vi "ADC Get Capabilities.vi"(7 "Initialize HW? (False)":bool, 8 "error in":errorcluster, 10 "parameters":T1, 11 "adc session in":T4={"niScope"={"channel cfg"=[], "sessions"=[], "multi cards"=FALSE, "channels"=0, "type"=enum."n/a", "memory [B/chn]"=0, "ext. clock [Hz]"=0.0, "samples count"=0, "use streaming"=FALSE, "proc setup"={"packet size [smpl]"=0, "current timeout [s]"=0.0, "blk2blk timeout [s]"=0.0, "event time"=timestamp(0 s since 1904-01-01), "temp sampl T [s]"=0.0, "data queue"=refnum, "stop notifier"=refnum, "proc ref"=refnum}, "sample width [B]"=0, "ranges [V]"=[], "trigger setup"={"coupling"=1, "level [V]"=0.0, "slope"=0, "mode"=enum."Immediate"}, "fs [Hz]"=0.0, "bitres [bit]"=0}, "3458A"={"channels"=[], "sync unit"={"VISA"="", "type"=enum."Picotest U6200A"}, "awg unit"={"type"=enum."Agilent 331xxA to 332xxA", "VISA"="", "enable 10MHz ref"=FALSE}, "sync mode"=enum."MASTER-SLAVE, MASTER clocked by TIMER", "streaming mode"=FALSE, "idn mode"=enum."Auto", "sampling mode"=enum."DCV", "Ts [s]"=0.0, "sample memory [B]"=0, "proc setup"={"channel id"=0, "packet size [smpl]"=0, "current timeout [s]"=0.0, "blk2blk timeout [s]"=0.0, "event time"=timestamp(0 s since 1904-01-01), "stop notifier"=refnum, "data queues"=[], "proc refs"=[], "bus semaphore"=refnum}, "sample size [B]"=0, "sample count"=0, "aux data"={"channel id"=0, "valid?"=[], "gain [V]"=[], "timestamp [s]"=[], "Ts [s]"=0.0, "abs timestamp"=timestamp(0 s since 1904-01-01), "t [deg C]"=[]}, "ranges [V]"=[], "aperture [s]"=0.0, "LEVEL trigger"={"edge"=enum."POS", "level [V]"=0.0, "coupling"=enum."DC"}, "trigger mode"=enum."AUTO", "measure temp.?"=FALSE, "disp mesages"=[], "shared bus?"=FALSE, "disable display?"=FALSE, "aper mode"=enum."Manual", "aper rules"=[]}, "dsdll"={"dsdll"={"dsdll path"=path "", "dsdll handle"=[], "output devices"=[], "capture devices"=[]}, "channels"=0, "device id"=0, "channel idns"=[], "proc setup"={"packet size [smpl]"=0, "current timeout [s]"=0.0, "blk2blk timeout [s]"=0.0, "event time"=timestamp(0 s since 1904-01-01), "data queue"=refnum, "stop notifier"=refnum, "proc ref"=refnum}, "samples count"=0, "fs [Hz]"=0.0}, "type"=enum."niScope", "channel idn str"=[], "aux instr idn str"=[], "modified?"=FALSE, "simadc"={"channels"=[], "range [V]"=0.0, "Ts step [s]"=0.0, "time [s]"=0.0, "fs [Hz]"=0.0, "count"=0, "smpl offset"=0, "set count"=0, "bit res"=0}, "force rst?"=FALSE, "exit mode"=enum."Immediate reset", "exit dly"=0.0, "exit tmr"=timestamp(0 s since 1904-01-01), "busy?"=FALSE, "accessed?"=FALSE, "QuADC session"={"channel cfg"=[], "sessions"=[], "multi cards"=FALSE, "channels"=0, "type"=enum."n/a", "memory [B/chn]"=0, "ext. clock [Hz]"=0.0, "samples count"=0, "use streaming"=FALSE, "proc setup"={"packet size [smpl]"=0, "current timeout [s]"=0.0, "blk2blk timeout [s]"=0.0, "event time"=timestamp(0 s since 1904-01-01), "temp sampl T [s]"=0.0, "data queue"=refnum, "stop notifier"=refnum, "proc ref"=refnum}, "sample width [B]"=0, "ranges [V]"=[], "trigger setup"={"coupling"=1, "level [V]"=0.0, "slope"=0, "mode"=enum."Immediate"}, "fs [Hz]"=0.0, "bitres [bit]"=0}} {"QuADC session"."trigger setup"."level [V]" format="%.2f"; "QuADC session"."trigger setup"."coupling" items=["AC"=0, "DC"=1, "HF Reject"=3, "LF Reject"=4, "AC Plus HF Reject"=1001]; "QuADC session"."channel cfg"."Clock fr. (Hz)" min=0.0 format="%#_9p"; "QuADC session"."channel cfg"."Number of JJ" min=1; "QuADC session"."channel cfg"."Range [Vpk]" min=0.0; "QuADC session"."channel cfg"."Channel" min=0; "3458A"."channels"."Range [Vpk]" min=0.0; "niScope"."trigger setup"."level [V]" format="%.2f"; "niScope"."trigger setup"."coupling" items=["AC"=0, "DC"=1, "HF Reject"=3, "LF Reject"=4, "AC Plus HF Reject"=1001]; "niScope"."channel cfg"."Range [Vpk]" min=0.0; "niScope"."channel cfg"."Channel" min=0}) -> (0 "error out":errorcluster, 2 "capabilities":T2, 3 "adc session out":T4={"niScope"={"channel cfg"=[], "sessions"=[], "multi cards"=FALSE, "channels"=0, "type"=enum."n/a", "memory [B/chn]"=0, "ext. clock [Hz]"=0.0, "samples count"=0, "use streaming"=FALSE, "proc setup"={"packet size [smpl]"=0, "current timeout [s]"=0.0, "blk2blk timeout [s]"=0.0, "event time"=timestamp(0 s since 1904-01-01), "temp sampl T [s]"=0.0, "data queue"=refnum, "stop notifier"=refnum, "proc ref"=refnum}, "sample width [B]"=0, "ranges [V]"=[], "trigger setup"={"coupling"=1, "level [V]"=0.0, "slope"=0, "mode"=enum."Immediate"}, "fs [Hz]"=0.0, "bitres [bit]"=0}, "3458A"={"channels"=[], "sync unit"={"VISA"="", "type"=enum."Picotest U6200A"}, "awg unit"={"type"=enum."Agilent 331xxA to 332xxA", "VISA"="", "enable 10MHz ref"=FALSE}, "sync mode"=enum."MASTER-SLAVE, MASTER clocked by TIMER", "streaming mode"=FALSE, "idn mode"=enum."Auto", "sampling mode"=enum."DCV", "Ts [s]"=0.0, "sample memory [B]"=0, "proc setup"={"channel id"=0, "packet size [smpl]"=0, "current timeout [s]"=0.0, "blk2blk timeout [s]"=0.0, "event time"=timestamp(0 s since 1904-01-01), "stop notifier"=refnum, "data queues"=[], "proc refs"=[], "bus semaphore"=refnum}, "sample size [B]"=0, "sample count"=0, "aux data"={"channel id"=0, "valid?"=[], "gain [V]"=[], "timestamp [s]"=[], "Ts [s]"=0.0, "abs timestamp"=timestamp(0 s since 1904-01-01), "t [deg C]"=[]}, "ranges [V]"=[], "aperture [s]"=0.0, "LEVEL trigger"={"edge"=enum."POS", "level [V]"=0.0, "coupling"=enum."DC"}, "trigger mode"=enum."AUTO", "measure temp.?"=FALSE, "disp mesages"=[], "shared bus?"=FALSE, "disable display?"=FALSE, "aper mode"=enum."Manual", "aper rules"=[]}, "dsdll"={"dsdll"={"dsdll path"=path "", "dsdll handle"=[], "output devices"=[], "capture devices"=[]}, "channels"=0, "device id"=0, "channel idns"=[], "proc setup"={"packet size [smpl]"=0, "current timeout [s]"=0.0, "blk2blk timeout [s]"=0.0, "event time"=timestamp(0 s since 1904-01-01), "data queue"=refnum, "stop notifier"=refnum, "proc ref"=refnum}, "samples count"=0, "fs [Hz]"=0.0}, "type"=enum."niScope", "channel idn str"=[], "aux instr idn str"=[], "modified?"=FALSE, "simadc"={"channels"=[], "range [V]"=0.0, "Ts step [s]"=0.0, "time [s]"=0.0, "fs [Hz]"=0.0, "count"=0, "smpl offset"=0, "set count"=0, "bit res"=0}, "force rst?"=FALSE, "exit mode"=enum."Immediate reset", "exit dly"=0.0, "exit tmr"=timestamp(0 s since 1904-01-01), "busy?"=FALSE, "accessed?"=FALSE, "QuADC session"={"channel cfg"=[], "sessions"=[], "multi cards"=FALSE, "channels"=0, "type"=enum."n/a", "memory [B/chn]"=0, "ext. clock [Hz]"=0.0, "samples count"=0, "use streaming"=FALSE, "proc setup"={"packet size [smpl]"=0, "current timeout [s]"=0.0, "blk2blk timeout [s]"=0.0, "event time"=timestamp(0 s since 1904-01-01), "temp sampl T [s]"=0.0, "data queue"=refnum, "stop notifier"=refnum, "proc ref"=refnum}, "sample width [B]"=0, "ranges [V]"=[], "trigger setup"={"coupling"=1, "level [V]"=0.0, "slope"=0, "mode"=enum."Immediate"}, "fs [Hz]"=0.0, "bitres [bit]"=0}} {"QuADC session"."trigger setup"."level [V]" format="%.2f"; "QuADC session"."trigger setup"."coupling" items=["AC"=0, "DC"=1, "HF Reject"=3, "LF Reject"=4, "AC Plus HF Reject"=1001]; "QuADC session"."channel cfg"."Clock fr. (Hz)" min=0.0 format="%#_9p"; "QuADC session"."channel cfg"."Number of JJ" min=1; "QuADC session"."channel cfg"."Range [Vpk]" min=0.0; "QuADC session"."channel cfg"."Channel" min=0; "3458A"."channels"."Range [Vpk]" min=0.0; "niScope"."trigger setup"."level [V]" format="%.2f"; "niScope"."trigger setup"."coupling" items=["AC"=0, "DC"=1, "HF Reject"=3, "LF Reject"=4, "AC Plus HF Reject"=1001]; "niScope"."channel cfg"."Range [Vpk]" min=0.0; "niScope"."channel cfg"."Channel" min=0})   [LabVIEW 2018]
doc: "This VI returns cluster of capabilities for selected HW. Note that to make it work the session must be either live (opened) or at least were opened and closed so the HW paramter data are in the session. Alternatively use option 'initialize HW'. That will open and close the HW so the data are read. Keep in mind this option may take some time so it should not be done every second in the GUI but for instance just once when GUI panel opens. Note that some of the paramters may not be valid if the input parameters are not assigned."
uses:
  ADC Session.ctl
  drivers/niScope/niScope Session.ctl
  drivers/niScope/niScope Virtual Channel Config.ctl
  drivers/niScope/niScope Virtual Channel Mode.ctl
  drivers/niScope/niScope Virtual Channel Input Z.ctl
  drivers/niScope/niScope Virtual Channel Coupling.ctl
  drivers/niScope/niScope Type.ctl
  drivers/niScope/niScope Digitizing Process Options.ctl
  drivers/niScope/niScope Data Packet.ctl
  drivers/niScope/niScope Trigger Setup.ctl
  <instrlib>/niScope/Controls/niScope trigger coupling.ctl
  <instrlib>/niScope/Controls/niScope trigger slope.ctl
  drivers/DMM/3458A Digitizer Session.ctl
  drivers/DMM/3458A Virtual Channel Config.ctl
  drivers/Counter/Counter Session.ctl
  drivers/Counter/Counter Type.ctl
  drivers/AWG/AWG Session.ctl
  drivers/AWG/AWG Type.ctl
  drivers/DMM/3458A Sync Mode.ctl
  drivers/DMM/3458A Idn Mode.ctl
  drivers/DMM/3458A Digitizing Low Levels/Configure/Sampling Mode.ctl
  drivers/DMM/3458A Digitizing Process Options.ctl
  drivers/DMM/3458A Data Packet.ctl
  drivers/DMM/3458A Aux Record Data.ctl
  drivers/DMM/3458A Digitizing Low Levels/Configure/Level Setup.ctl
  drivers/DMM/3458A Digitizing Low Levels/Configure/First Sample Trigger.ctl
  drivers/DMM/3458A Aperture Selection Mode.ctl
  drivers/dsdll/DSDLL Session.ctl
  drivers/dsdll/dsdll source distribution/dsdll_instance.ctl
  drivers/dsdll/dsdll source distribution/dsdll_device_record.ctl
  drivers/dsdll/DSDLL Process Config.ctl
  drivers/dsdll/DSDLL Data Packet.ctl
  ADC Type.ctl
  drivers/simulated_adc/SimAdc Config.ctl
  drivers/simulated_adc/SimAdc Channel Cfg.ctl
  ADC On Close Action.ctl
  drivers/Quatsch_driver/QuADCDriver/QuADC Session.ctl
  drivers/Quatsch_driver/QuADCDriver/QuADC Virtual Channel Config.ctl
  drivers/Quatsch_driver/QuADCDriver/QuADC Virtual Channel Mode.ctl
  drivers/Quatsch_driver/QuADCDriver/QuADC Virtual Channel Input Z.ctl
  drivers/Quatsch_driver/QuADCDriver/QuADC Virtual Channel Coupling.ctl
  drivers/Quatsch_driver/QuADCDriver/QuADC Type.ctl
  drivers/Quatsch_driver/QuADCDriver/QuADC Digitizing Process Options.ctl
  drivers/Quatsch_driver/QuADCDriver/QuADC Data Packet.ctl
  drivers/Quatsch_driver/QuADCDriver/QuADC Trigger Setup.ctl
  ADC Capabilities.ctl
  ADC Sampling Rate Step Mode.ctl
  ADC Capabilities Parameters.ctl
  drivers/niScope/niScope Virtual Digitizer.lvlib
  drivers/DMM/3458A Virtual Digitizer.lvlib
  drivers/Quatsch_driver/QuADCDriver/QuADC Virtual Digitizer.lvlib
  drivers/Counter/Counter.lvlib
  drivers/AWG/AWG.lvlib
  drivers/DMM/3458A Digitizing Low Levels/3458A Digitizing Low Levels.lvlib
  drivers/dsdll/DSDLL Virtual Digitizer.lvlib
  drivers/dsdll/dsdll source distribution/dsdll.lvlib
panel:
  # "IP Address"
  # "."
  # "."
  # "."
  # ":"
  # "IP Address"
  # "."
  # "."
  # "."
  # ":"
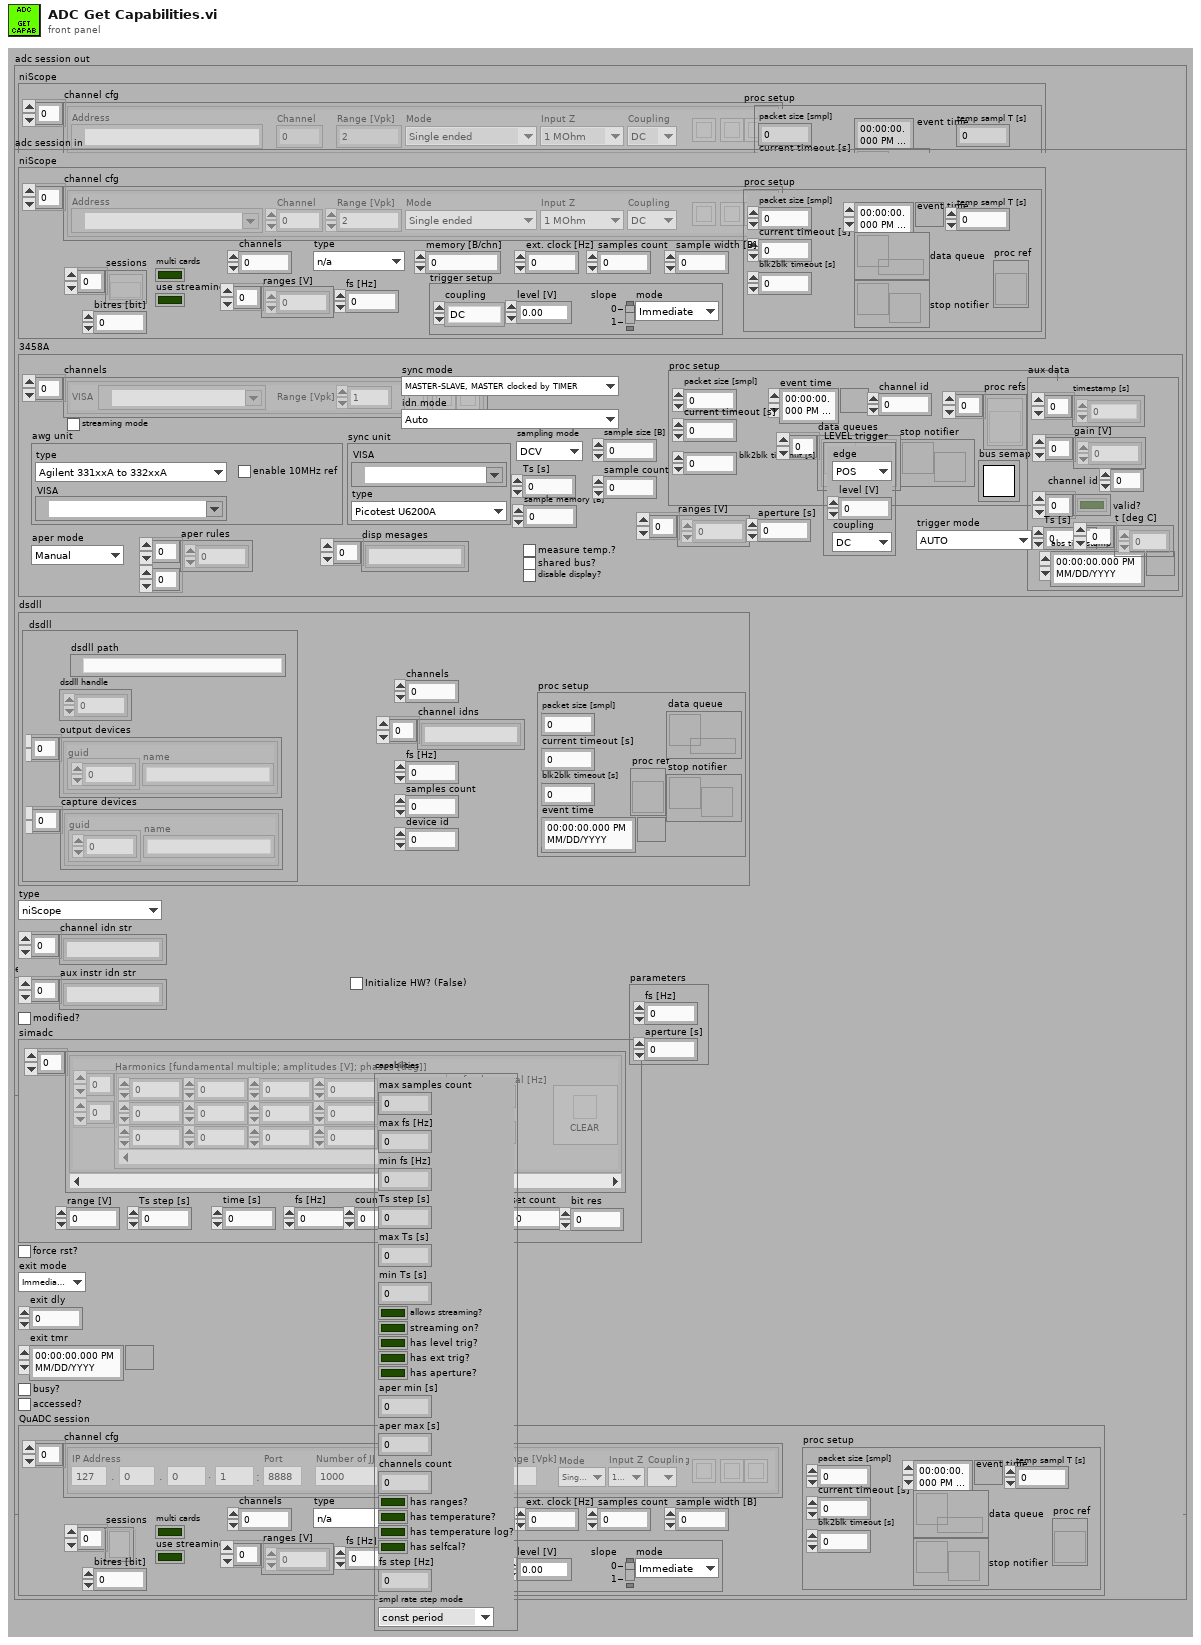
[diagram p1: front panel]
types:
  T1 = typedef "ADC Capabilities Parameters.ctl" = cluster{"fs [Hz]":dbl, "aperture [s]":dbl}
  T2 = typedef "ADC Capabilities.ctl" = cluster{"max samples count":i64, "max fs [Hz]":ext, "min fs [Hz]":ext, "Ts step [s]":ext, "max Ts [s]":ext, "min Ts [s]":ext, "allows streaming?":bool, "streaming on?":bool, "has level trig?":bool, "has ext trig?":bool, "has aperture?":bool, "aper min [s]":dbl, "aper max [s]":dbl, "channels count":i32, "has ranges?":bool, "has temperature?":bool, "has temperature log?":bool, "has selfcal?":bool, "fs step [Hz]":ext, "smpl rate step mode":T3}
  T3 = typedef "ADC Sampling Rate Step Mode.ctl" = enum16{"const period", "const frequency"}
  T4 = typedef "ADC Session.ctl" = cluster{"niScope":T5, "3458A":T15, "dsdll":T30, "type":T34, "channel idn str":string[], "aux instr idn str":string[], "modified?":bool, "simadc":T35, "force rst?":bool, "exit mode":T37, "exit dly":dbl, "exit tmr":timestamp, "busy?":bool, "accessed?":bool, "QuADC session":T38}
  T5 = typedef "niScope Virtual Digitizer.lvlib/niScope Session.ctl" = cluster{"channel cfg":T6[], "sessions":refnum<k20>[], "multi cards":bool, "channels":i32, "type":T10, "memory [B/chn]":i32, "ext. clock [Hz]":dbl, "samples count":i64, "use streaming":bool, "proc setup":T11, "sample width [B]":i32, "ranges [V]":dbl[], "trigger setup":T12, "fs [Hz]":dbl, "bitres [bit]":i32}
  T6 = typedef "niScope Virtual Digitizer.lvlib/niScope Virtual Channel Config.ctl" = cluster{"Address":refnum<k15>, "Channel":i32, "Mode":T7, "Input Z":T8, "Coupling":T9, "Range [Vpk]":dbl, "btn clr":bool, "btn up":bool, "btn down":bool}
  T7 = typedef "niScope Virtual Digitizer.lvlib/niScope Virtual Channel Mode.ctl" = enum16{"Single ended", "Unbal. differential", "Differential"}
  T8 = typedef "niScope Virtual Digitizer.lvlib/niScope Virtual Channel Input Z.ctl" = enum16{"1 MOhm", "50 Ohm"}
  T9 = typedef "niScope Virtual Digitizer.lvlib/niScope Virtual Channel Coupling.ctl" = enum16{"AC", "DC", "GND"}
  T10 = typedef "niScope Virtual Digitizer.lvlib/niScope Type.ctl" = enum16{"n/a", "5922"}
  T11 = typedef "niScope Virtual Digitizer.lvlib/niScope Digitizing Process Options.ctl" = cluster{"packet size [smpl]":i64, "current timeout [s]":dbl, "blk2blk timeout [s]":dbl, "event time":timestamp, "temp sampl T [s]":dbl, "data queue":refnum<queue>, "stop notifier":refnum<notifier>, "proc ref":refnum<vi>}
  T12 = typedef "niScope Virtual Digitizer.lvlib/niScope Trigger Setup.ctl" = cluster{"coupling":T13, "level [V]":dbl, "slope":T14, "mode":enum16{"Immediate", "External", "Level"}}
  T13 = typedef "niScope trigger coupling.ctl" = u16
  T14 = typedef "niScope trigger slope.ctl" = i32
  T15 = typedef "3458A Virtual Digitizer.lvlib/3458A Digitizer Session.ctl" = cluster{"channels":T16[], "sync unit":T17, "awg unit":T19, "sync mode":T21, "streaming mode":bool, "idn mode":T22, "sampling mode":T23, "Ts [s]":dbl, "sample memory [B]":i32, "proc setup":T24, "sample size [B]":i32, "sample count":i32, "aux data":T26, "ranges [V]":dbl[], "aperture [s]":dbl, "LEVEL trigger":T27, "trigger mode":T28, "measure temp.?":bool, "disp mesages":string[], "shared bus?":bool, "disable display?":bool, "aper mode":T29, "aper rules":dbl[][]}
  T16 = typedef "3458A Virtual Digitizer.lvlib/3458A Virtual Channel Config.ctl" = cluster{"VISA":refnum<visa-resource-name>, "Range [Vpk]":dbl, "btn clr":bool, "btn up":bool, "btn down":bool}
  T17 = typedef "Counter.lvlib/Counter Session.ctl" = cluster{"VISA":refnum<visa-resource-name>, "type":T18}
  T18 = typedef "Counter.lvlib/Counter Type.ctl" = enum16{"Picotest U6200A", "dummy"}
  T19 = typedef "AWG.lvlib/AWG Session.ctl" = cluster{"type":T20, "VISA":refnum<visa-resource-name>, "enable 10MHz ref":bool}
  T20 = typedef "AWG.lvlib/AWG Type.ctl" = enum16{"Agilent 331xxA to 332xxA", "Agilent 335xxA to 336xxA", "Tektronix AFG3101C", "dummy"}
  T21 = typedef "3458A Virtual Digitizer.lvlib/3458A Sync Mode.ctl" = enum16{"MASTER-SLAVE, MASTER clocked by TIMER", "MASTER-SLAVE, MASTER clocked by AWG", "ALL clocked by AWG", "MASTER-SLAVE, ALL clocked by TIMER", "ALL clocked by AWG with DFLL"}
  T22 = typedef "3458A Virtual Digitizer.lvlib/3458A Idn Mode.ctl" = enum16{"Auto", "Sequential (chn A, chn B, ...)", "From calibration string"}
  T23 = typedef "3458A Virtual Digitizer.lvlib/3458A Digitizing Low Levels.lvlib/Sampling Mode.ctl" = enum16{"DCV", "DSDC", "DSAC"}
  T24 = typedef "3458A Virtual Digitizer.lvlib/3458A Digitizing Process Options.ctl" = cluster{"channel id":i32, "packet size [smpl]":i32, "current timeout [s]":dbl, "blk2blk timeout [s]":dbl, "event time":timestamp, "stop notifier":refnum<notifier>, "data queues":refnum<queue>[], "proc refs":refnum<vi>[], "bus semaphore":T25}
  T25 = typedef "Semaphore RefNum" = refnum<k1>
  T26 = typedef "3458A Virtual Digitizer.lvlib/3458A Aux Record Data.ctl" = cluster{"channel id":i32, "valid?":bool[], "gain [V]":dbl[], "timestamp [s]":dbl[], "Ts [s]":dbl, "abs timestamp":timestamp, "t [deg C]":dbl[]}
  T27 = typedef "3458A Virtual Digitizer.lvlib/3458A Digitizing Low Levels.lvlib/Level Setup.ctl" = cluster{"edge":enum16{"POS", "NEG"}, "level [V]":dbl, "coupling":enum16{"DC", "AC"}}
  T28 = typedef "3458A Virtual Digitizer.lvlib/3458A Digitizing Low Levels.lvlib/First Sample Trigger.ctl" = enum16{"AUTO", "EXT", "SYN", "SGL", "HOLD", "LEVEL"}
  T29 = typedef "3458A Virtual Digitizer.lvlib/3458A Aperture Selection Mode.ctl" = enum16{"Manual", "Maximum", "Table"}
  T30 = typedef "DSDLL Virtual Digitizer.lvlib/DSDLL Session.ctl" = cluster{"dsdll":T31, "channels":i32, "device id":i32, "channel idns":string[], "proc setup":T33, "samples count":i32, "fs [Hz]":dbl}
  T31 = typedef "dsdll.lvlib/dsdll_instance.ctl" = cluster{"dsdll path":path, "dsdll handle":u8[], "output devices":T32[], "capture devices":T32[]}
  T32 = typedef "dsdll.lvlib/dsdll_device_record.ctl" = cluster{"guid":u8[], "name":string}
  T33 = typedef "DSDLL Virtual Digitizer.lvlib/DSDLL Process Config.ctl" = cluster{"packet size [smpl]":i32, "current timeout [s]":dbl, "blk2blk timeout [s]":dbl, "event time":timestamp, "data queue":refnum<queue>, "stop notifier":refnum<notifier>, "proc ref":refnum<vi>}
  T34 = typedef "ADC Type.ctl" = enum16{"niScope", "3458A", "DirectSound DLL", "dummy", "QuADC"}
  T35 = typedef "SimAdc Config.ctl" = cluster{"channels":T36[], "range [V]":dbl, "Ts step [s]":dbl, "time [s]":dbl, "fs [Hz]":dbl, "count":i64, "smpl offset":i64, "set count":i64, "bit res":i32}
  T36 = typedef "SimAdc Channel Cfg.ctl" = cluster{"harmonics":dbl[][], "btn clear":bool, "noise":dbl, "fundamental [Hz]":dbl}
  T37 = typedef "ADC On Close Action.ctl" = enum16{"Immediate reset", "Delayed reset"}
  T38 = typedef "QuADC Virtual Digitizer.lvlib/QuADC Session.ctl" = cluster{"channel cfg":T39[], "sessions":refnum<k5>[], "multi cards":bool, "channels":i32, "type":T43, "memory [B/chn]":i32, "ext. clock [Hz]":dbl, "samples count":i64, "use streaming":bool, "proc setup":T44, "sample width [B]":i32, "ranges [V]":dbl[], "trigger setup":T45, "fs [Hz]":dbl, "bitres [bit]":i32}
  T39 = typedef "QuADC Virtual Digitizer.lvlib/QuADC Virtual Channel Config.ctl" = cluster{"Channel":i32, "Mode":T40, "Input Z":T41, "Coupling":T42, "Range [Vpk]":dbl, "btn clr":bool, "btn up":bool, "btn down":bool, "IP address A":u8, "IP address B":u8, "IP address C":u8, "IP address D":u8, "Port":u16, "Number of JJ":u32, "Clock fr. (Hz)":dbl}
  T40 = typedef "QuADC Virtual Digitizer.lvlib/QuADC Virtual Channel Mode.ctl" = enum16{"Single ended", "Unbal. differential", "Differential"}
  T41 = typedef "QuADC Virtual Digitizer.lvlib/QuADC Virtual Channel Input Z.ctl" = enum16{"1 MOhm", "50 Ohm"}
  T42 = typedef "QuADC Virtual Digitizer.lvlib/QuADC Virtual Channel Coupling.ctl" = enum16{"AC", "DC", "GND"}
  T43 = typedef "QuADC Virtual Digitizer.lvlib/QuADC Type.ctl" = enum16{"n/a", "v1"}
  T44 = typedef "QuADC Virtual Digitizer.lvlib/QuADC Digitizing Process Options.ctl" = cluster{"packet size [smpl]":i64, "current timeout [s]":dbl, "blk2blk timeout [s]":dbl, "event time":timestamp, "temp sampl T [s]":dbl, "data queue":refnum<queue>, "stop notifier":refnum<notifier>, "proc ref":refnum<vi>}
  T45 = typedef "QuADC Virtual Digitizer.lvlib/QuADC Trigger Setup.ctl" = cluster{"coupling":T13, "level [V]":dbl, "slope":T14, "mode":enum16{"Immediate", "External", "Level"}}
  T46 = typedef "3458A Virtual Digitizer.lvlib/3458A Capabilities.ctl" = cluster{"max samples count":i64, "max fs [Hz]":ext, "min fs [Hz]":ext, "Ts step [s]":ext, "max Ts [s]":ext, "min Ts [s]":ext, "allows streaming?":bool, "streaming on?":bool, "has level trig?":bool, "has ext trig?":bool, "min aperture [s]":dbl, "max aperture [s]":dbl, "has aperture?":bool, "channels count":i32, "has temp.?":bool, "fs step [Hz]":ext, "const fs step?":bool}
  T47 = typedef "niScope Virtual Digitizer.lvlib/niScope Capabilities.ctl" = cluster{"max samples count":i64, "max fs [Hz]":ext, "min fs [Hz]":ext, "Ts step [s]":ext, "max Ts [s]":ext, "min Ts [s]":ext, "allows streaming?":bool, "streaming on?":bool, "has level trig?":bool, "has ext trig?":bool, "channels count":i32, "has ranges?":bool}
  T48 = typedef "QuADC Virtual Digitizer.lvlib/QuADC Capabilities.ctl" = cluster{"max samples count":i64, "max fs [Hz]":ext, "min fs [Hz]":ext, "Ts step [s]":ext, "max Ts [s]":ext, "min Ts [s]":ext, "allows streaming?":bool, "streaming on?":bool, "has level trig?":bool, "has ext trig?":bool, "channels count":i32, "has ranges?":bool}
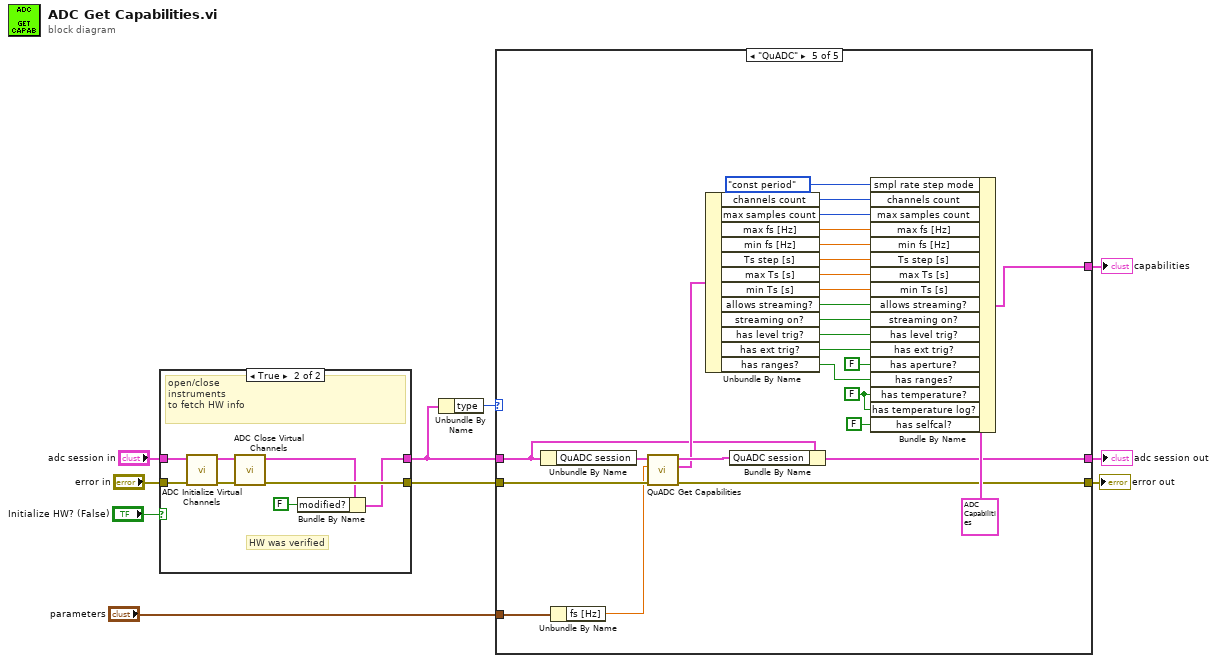
[diagram p0: block diagram]
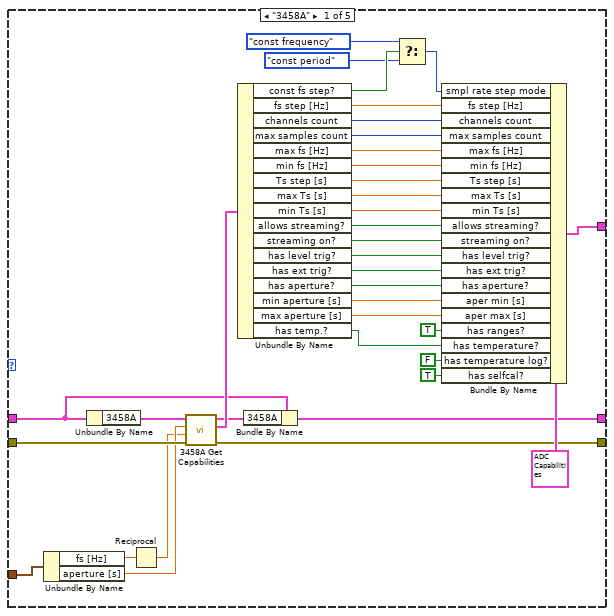
[diagram p2: hidden frame]
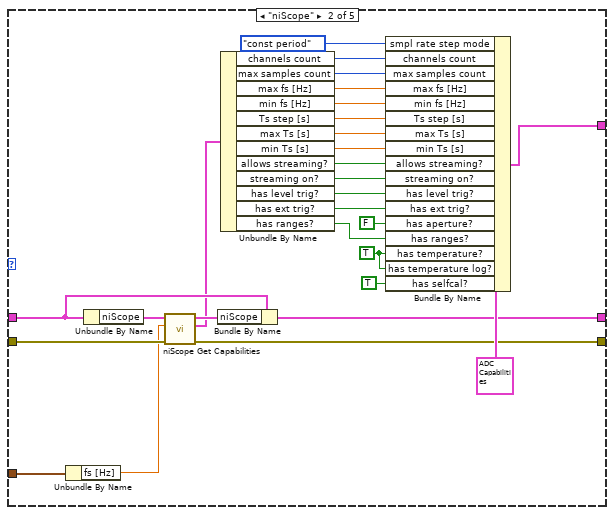
[diagram p3: hidden frame]
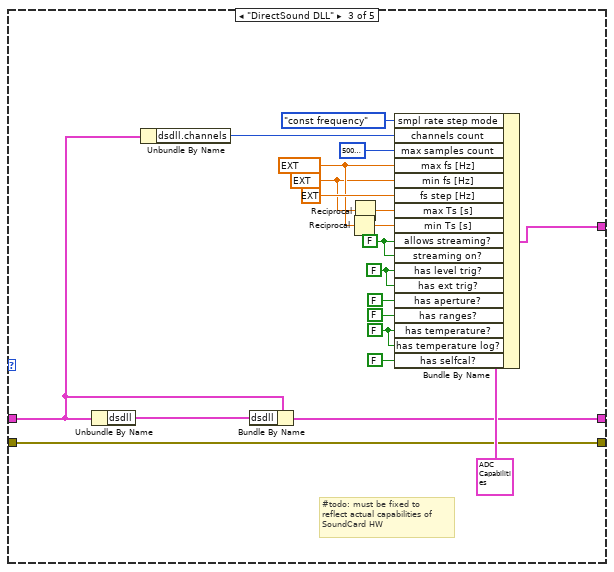
[diagram p4: hidden frame]
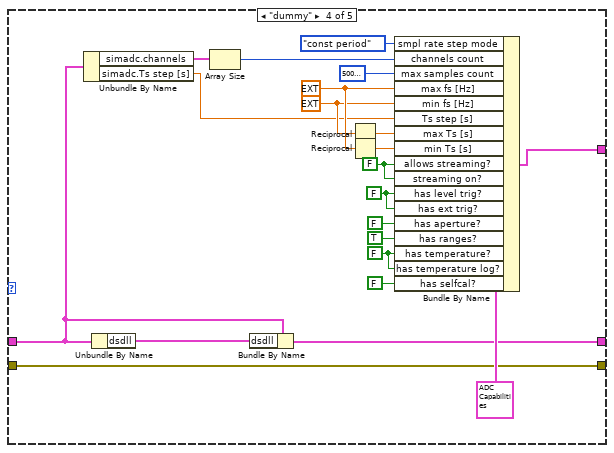
[diagram p5: hidden frame]
diagram:
  n1 = case shown="True" "Initialize HW? (False)" {
    tunnel: "error in" -> [w11 w20]
    tunnel: "adc session in" -> [w12 w17]
    tunnel: [w11 w16] -> w6
    tunnel: [w12 w15] -> w5
    frame False {
    }
    frame True {
      # "HW was verified"
      # "open/close\ninstruments\nto fetch HW info"
      n2 = call "ADC Initialize Virtual Channels.vi"("error in"=w20, "adc session in"=w17) -> ("error out"=w19:errorcluster, "adc session out"=w18:T4)  [unwired: 5 in, 3 out]
      n3 = call "ADC Close Virtual Channels.vi"("error in"=w19, "adc session in"=w18) -> ("error out"=w16:errorcluster, "adc session out"=w14:T4)  [unwired: 8 in]
      n4 = Bundle By Name(cluster=w14, "modified?"=FALSE) -> (w15:T4)
    }
  }
  n5 = Unbundle By Name(w5) -> ("type"=w7:T34)
  n6 = case shown="\"QuADC\"" w7 {
    tunnel: w6 -> [w56 w69 w88 w110 w130]
    tunnel: w5 -> [w41 w71 w98 w119 w125]
    tunnel: [w42 w65 w88 w110 w131] -> w4
    tunnel: [w39 w70 w101 w122 w133] -> w3
    tunnel: [w38 w64 w100 w121 w132] -> w2
    tunnel: "parameters" -> [w37 w63 _ _ w134]
    frame "3458A" {
      n7 = Unbundle By Name(w37) -> ("fs [Hz]"=w32:dbl, "aperture [s]"=w36:dbl)
      n8 = Unbundle By Name(w41) -> ("3458A"=w55:T15)
      n9 = Reciprocal(x=w32) -> (1/x=w31:dbl)
      n10 = call "3458A Get Capabilities.vi"("error in"=w56, "Ts [s]"=w31, "aperture [s]"=w36, "digitizer session in"=w55) -> ("error out"=w42:errorcluster, "capabilities"=w54:T46, "digitizer session out"=w40:T15)  [unwired: 5 in]
      n11 = Unbundle By Name(w54) -> ("const fs step?"=w23:bool, "fs step [Hz]"=w25:ext, "channels count"=w30:i32, "max samples count"=w52:i64, "max fs [Hz]"=w51:ext, "min fs [Hz]"=w50:ext, "Ts step [s]"=w49:ext, "max Ts [s]"=w48:ext, "min Ts [s]"=w47:ext, "allows streaming?"=w46:bool, "streaming on?"=w45:bool, "has level trig?"=w44:bool, "has ext trig?"=w43:bool, "has aperture?"=w35:bool, "min aperture [s]"=w34:dbl, "max aperture [s]"=w33:dbl, "has temp.?"=w27:bool)
      n12 = Bundle By Name(cluster=w41, "3458A"=w40) -> (w39:T4)
      n13 = Select(t=ADC_Sampling_Rate_Step_Mode."const frequency" ("smpl rate step mode"), s=w23, f=ADC_Sampling_Rate_Step_Mode."const period" ("smpl rate step mode")) -> (s? t:f=w24:T3)
      n14 = Bundle By Name(cluster=T2 {"max samples count"=0, "max fs [Hz]"=0.0, "min fs [Hz]"=0.0, "Ts step [s]"=0.0, "max Ts [s]"=0.0, "min Ts [s]"=0.0, "allows streaming?"=FALSE, "streaming on?"=FALSE, "has level trig?"=FALSE, "has ext trig?"=FALSE, "has aperture?"=FALSE, "aper min [s]"=0.0, "aper max [s]"=0.0, "channels count"=0, "has ranges?"=FALSE, "has temperature?"=FALSE, "has temperature log?"=FALSE, "has selfcal?"=FALSE, "fs step [Hz]"=0.0, "smpl rate step mode"=enum."const period"} ("capabilities"), "smpl rate step mode"=w24, "fs step [Hz]"=w25, "channels count"=w30, "max samples count"=w52, "max fs [Hz]"=w51, "min fs [Hz]"=w50, "Ts step [s]"=w49, "max Ts [s]"=w48, "min Ts [s]"=w47, "allows streaming?"=w46, "streaming on?"=w45, "has level trig?"=w44, "has ext trig?"=w43, "has aperture?"=w35, "aper min [s]"=w34, "aper max [s]"=w33, "has ranges?"=TRUE, "has temperature?"=w27, "has temperature log?"=FALSE, "has selfcal?"=TRUE) -> (w38:T2)
    }
    frame "niScope" {
      w59 = TRUE ("has temperature?")
      n15 = Unbundle By Name(w63) -> ("fs [Hz]"=w62:dbl)
      n16 = Unbundle By Name(w71) -> ("niScope"=w68:T5)
      n17 = call "niScope Get Capabilities.vi"("error in"=w69, "fs [Hz]"=w62, "niScope session in"=w68) -> ("error out"=w65:errorcluster, "capabilities"=w66:T47, "niScope session out"=w67:T5)  [unwired: 6 in]
      n18 = Bundle By Name(cluster=w71, "niScope"=w67) -> (w70:T4)
      n19 = Unbundle By Name(w66) -> ("channels count"=w61:i32, "max samples count"=w82:i64, "max fs [Hz]"=w81:ext, "min fs [Hz]"=w80:ext, "Ts step [s]"=w79:ext, "max Ts [s]"=w78:ext, "min Ts [s]"=w77:ext, "allows streaming?"=w76:bool, "streaming on?"=w75:bool, "has level trig?"=w74:bool, "has ext trig?"=w73:bool, "has ranges?"=w60:bool)
      n20 = Bundle By Name(cluster=T2 {"max samples count"=0, "max fs [Hz]"=0.0, "min fs [Hz]"=0.0, "Ts step [s]"=0.0, "max Ts [s]"=0.0, "min Ts [s]"=0.0, "allows streaming?"=FALSE, "streaming on?"=FALSE, "has level trig?"=FALSE, "has ext trig?"=FALSE, "has aperture?"=FALSE, "aper min [s]"=0.0, "aper max [s]"=0.0, "channels count"=0, "has ranges?"=FALSE, "has temperature?"=FALSE, "has temperature log?"=FALSE, "has selfcal?"=FALSE, "fs step [Hz]"=0.0, "smpl rate step mode"=enum."const period"} ("capabilities"), "smpl rate step mode"=ADC_Sampling_Rate_Step_Mode."const period", "channels count"=w61, "max samples count"=w82, "max fs [Hz]"=w81, "min fs [Hz]"=w80, "Ts step [s]"=w79, "max Ts [s]"=w78, "min Ts [s]"=w77, "allows streaming?"=w76, "streaming on?"=w75, "has level trig?"=w74, "has ext trig?"=w73, "has aperture?"=FALSE, "has ranges?"=w60, "has temperature?"=w59, "has temperature log?"=w59, "has selfcal?"=TRUE) -> (w64:T2)
    }
    frame "DirectSound DLL" {
      w86 = FALSE ("has temperature?")
      w89 = FALSE ("has level trig?")
      w90 = FALSE ("allows streaming?")
      w91 = ext 8000.0 ("min fs [Hz]")
      w94 = ext 192000.0 ("max fs [Hz]")
      # "#todo: must be fixed to \nreflect actual capabilities of\nSoundCard HW"
      n21 = Unbundle By Name(w98) -> ("dsdll"=w99:T30)
      n22 = Unbundle By Name(w98) -> ("dsdll.channels"=w97:i32)
      n23 = Bundle By Name(cluster=w98, "dsdll"=w99) -> (w101:T4)
      n24 = Reciprocal(x=w94) -> (1/x=w93:ext)
      n25 = Reciprocal(x=w91) -> (1/x=w92:ext)
      n26 = Bundle By Name(cluster=T2 {"max samples count"=0, "max fs [Hz]"=0.0, "min fs [Hz]"=0.0, "Ts step [s]"=0.0, "max Ts [s]"=0.0, "min Ts [s]"=0.0, "allows streaming?"=FALSE, "streaming on?"=FALSE, "has level trig?"=FALSE, "has ext trig?"=FALSE, "has aperture?"=FALSE, "aper min [s]"=0.0, "aper max [s]"=0.0, "channels count"=0, "has ranges?"=FALSE, "has temperature?"=FALSE, "has temperature log?"=FALSE, "has selfcal?"=FALSE, "fs step [Hz]"=0.0, "smpl rate step mode"=enum."const period"} ("capabilities"), "smpl rate step mode"=ADC_Sampling_Rate_Step_Mode."const frequency", "channels count"=w97, "max samples count"=50000000, "max fs [Hz]"=w94, "min fs [Hz]"=w91, "fs step [Hz]"=ext 1.0 ("Ts step [s]"), "max Ts [s]"=w92, "min Ts [s]"=w93, "allows streaming?"=w90, "streaming on?"=w90, "has level trig?"=w89, "has ext trig?"=w89, "has aperture?"=FALSE, "has ranges?"=FALSE, "has temperature?"=w86, "has temperature log?"=w86, "has selfcal?"=FALSE) -> (w100:T2)
    }
    frame "dummy" {
      w108 = FALSE ("has temperature?")
      w111 = FALSE ("has level trig?")
      w112 = FALSE ("allows streaming?")
      w113 = ext 1.0 ("min fs [Hz]")
      w116 = ext 1000000000.0 ("max fs [Hz]")
      n27 = Unbundle By Name(w119) -> ("simadc.channels"=w118:T36[], "simadc.Ts step [s]"=w105:dbl)
      n28 = Unbundle By Name(w119) -> ("dsdll"=w120:T30)
      n29 = Array Size(array=w118) -> (size(s)=w106:i32)
      n30 = Bundle By Name(cluster=w119, "dsdll"=w120) -> (w122:T4)
      n31 = Reciprocal(x=w113) -> (1/x=w114:ext)
      n32 = Reciprocal(x=w116) -> (1/x=w115:ext)
      n33 = Bundle By Name(cluster=T2 {"max samples count"=0, "max fs [Hz]"=0.0, "min fs [Hz]"=0.0, "Ts step [s]"=0.0, "max Ts [s]"=0.0, "min Ts [s]"=0.0, "allows streaming?"=FALSE, "streaming on?"=FALSE, "has level trig?"=FALSE, "has ext trig?"=FALSE, "has aperture?"=FALSE, "aper min [s]"=0.0, "aper max [s]"=0.0, "channels count"=0, "has ranges?"=FALSE, "has temperature?"=FALSE, "has temperature log?"=FALSE, "has selfcal?"=FALSE, "fs step [Hz]"=0.0, "smpl rate step mode"=enum."const period"} ("capabilities"), "smpl rate step mode"=ADC_Sampling_Rate_Step_Mode."const period", "channels count"=w106, "max samples count"=50000000, "max fs [Hz]"=w116, "min fs [Hz]"=w113, "Ts step [s]"=w105, "max Ts [s]"=w114, "min Ts [s]"=w115, "allows streaming?"=w112, "streaming on?"=w112, "has level trig?"=w111, "has ext trig?"=w111, "has aperture?"=FALSE, "has ranges?"=TRUE, "has temperature?"=w108, "has temperature log?"=w108, "has selfcal?"=FALSE) -> (w121:T2)
    }
    frame "QuADC" {
      w137 = FALSE ("has temperature?")
      n34 = Unbundle By Name(w125) -> ("QuADC session"=w128:T38)
      n35 = Unbundle By Name(w134) -> ("fs [Hz]"=w129:dbl)
      n36 = call "QuADC Get Capabilities.vi"("error in"=w130, "fs [Hz]"=w129, "QuADC session in"=w128) -> ("error out"=w131:errorcluster, "capabilities"=w126:T48, "QuADC session out"=w127:T38)  [unwired: 6 in]
      n37 = Unbundle By Name(w126) -> ("channels count"=w139:i32, "max samples count"=w150:i64, "max fs [Hz]"=w149:ext, "min fs [Hz]"=w148:ext, "Ts step [s]"=w147:ext, "max Ts [s]"=w146:ext, "min Ts [s]"=w145:ext, "allows streaming?"=w144:bool, "streaming on?"=w143:bool, "has level trig?"=w142:bool, "has ext trig?"=w141:bool, "has ranges?"=w138:bool)
      n38 = Bundle By Name(cluster=w125, "QuADC session"=w127) -> (w133:T4)
      n39 = Bundle By Name(cluster=T2 {"max samples count"=0, "max fs [Hz]"=0.0, "min fs [Hz]"=0.0, "Ts step [s]"=0.0, "max Ts [s]"=0.0, "min Ts [s]"=0.0, "allows streaming?"=FALSE, "streaming on?"=FALSE, "has level trig?"=FALSE, "has ext trig?"=FALSE, "has aperture?"=FALSE, "aper min [s]"=0.0, "aper max [s]"=0.0, "channels count"=0, "has ranges?"=FALSE, "has temperature?"=FALSE, "has temperature log?"=FALSE, "has selfcal?"=FALSE, "fs step [Hz]"=0.0, "smpl rate step mode"=enum."const period"} ("capabilities"), "smpl rate step mode"=ADC_Sampling_Rate_Step_Mode."const period", "channels count"=w139, "max samples count"=w150, "max fs [Hz]"=w149, "min fs [Hz]"=w148, "Ts step [s]"=w147, "max Ts [s]"=w146, "min Ts [s]"=w145, "allows streaming?"=w144, "streaming on?"=w143, "has level trig?"=w142, "has ext trig?"=w141, "has aperture?"=FALSE, "has ranges?"=w138, "has temperature?"=w137, "has temperature log?"=w137, "has selfcal?"=FALSE) -> (w132:T2)
    }
  }
  "error out" <- w4
  "adc session out" <- w3
  "capabilities" <- w2
